vi "Get Descriptor.vi"(11 "output_actor in":refnum<class "Output Actor.lvclass">) -> (2 "Descriptor":string, 3 "output_actor out":refnum<class "Output Actor.lvclass">)   [LabVIEW 2015, in "Output Actor.lvclass"]
uses:
  Output Actor.lvclass
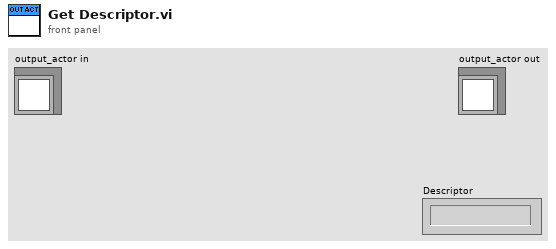
[diagram p1: front panel]
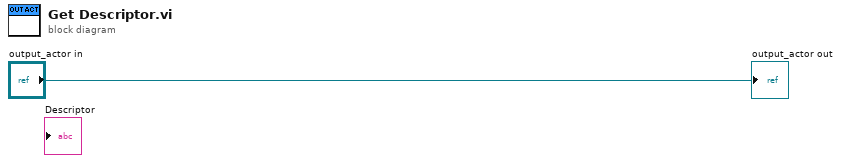
[diagram p0: block diagram]
diagram:
  "output_actor out" <- "output_actor in"
